vi "RelaySwitching.vi"() -> ()   [LabVIEW 2020]
uses:
  <vilib>/Instr/_visa.llb/VISA Configure Serial Port (Instr).vi
panel:
  in  "Boolean 3":bool
  in  "VISA resource name 3":refnum<visa-resource-name>
  in  "VISA resource name 2":refnum<visa-resource-name>
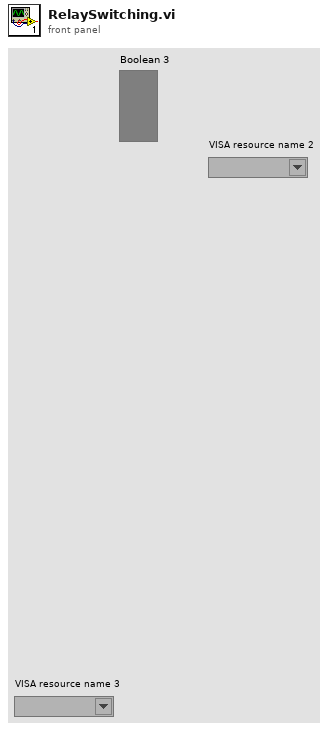
[diagram p1: front panel]
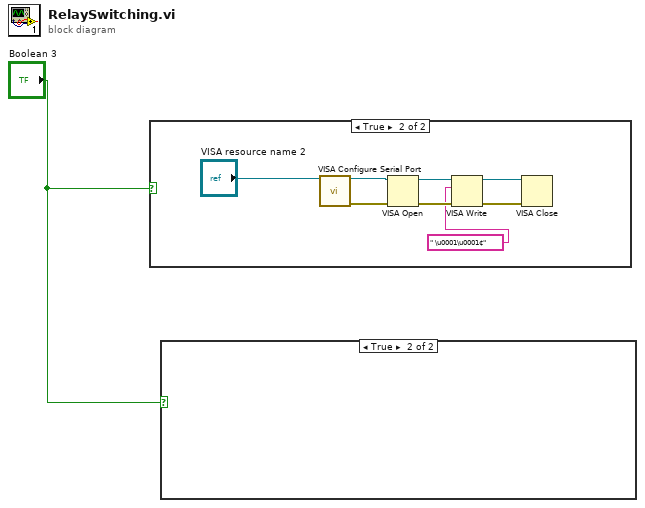
[diagram p0: block diagram]
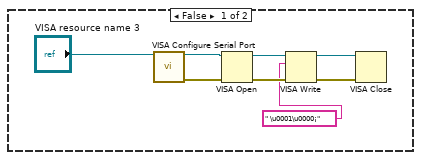
[diagram p2: hidden frame]
diagram:
  n1 = case shown="True" "Boolean 3" {
    frame False {
    }
    frame True {
      n2 = call-poly "VISA Configure Serial Port"("VISA resource name"="VISA resource name 2") -> ("VISA resource name out"=w9:refnum<visa-resource-name>, "error out"=w8:errorcluster)  [unwired: 13 in]
      n3 = VISA Open(error in (no error)=w8, VISA resource name=w9) -> (VISA resource name=w7:refnum<visa-resource-name>, error out=w6:errorcluster)  [unwired: 3 in]
      n4 = VISA Write(VISA resource name=w7, write buffer=" \u0001\u0001¢", error in (no error)=w6) -> (VISA resource name out=w5:refnum<visa-resource-name>, error out=w4:errorcluster)  [unwired: 1 out]
      n5 = VISA Close(VISA resource name=w5, error in (no error)=w4) -> ()  [unwired: 1 out]
    }
  }
  n6 = case shown="True" "Boolean 3" {
    frame False {
      n7 = call-poly "VISA Configure Serial Port"("VISA resource name"="VISA resource name 3") -> ("VISA resource name out"=w17:refnum<visa-resource-name>, "error out"=w16:errorcluster)  [unwired: 13 in]
      n8 = VISA Open(error in (no error)=w16, VISA resource name=w17) -> (VISA resource name=w15:refnum<visa-resource-name>, error out=w14:errorcluster)  [unwired: 3 in]
      n9 = VISA Write(VISA resource name=w15, write buffer=" \u0001\u0000¡", error in (no error)=w14) -> (VISA resource name out=w13:refnum<visa-resource-name>, error out=w12:errorcluster)  [unwired: 1 out]
      n10 = VISA Close(VISA resource name=w13, error in (no error)=w12) -> ()  [unwired: 1 out]
    }
    frame True {
    }
  }
